vi "Solve Tridiagonal Equations (multiple right hand DBL).vi"(8 "Known Matrix":T1, 9 "Pivot":i32[](array[numeric]), 10 "U":T2, 11 "L":dbl[](array[numeric])) -> (0 "error":i32, 3 "Solution Matrix":T1)   [LabVIEW 2020, in "NI_AALPro.lvlib"]
uses:
  NI_AALPro.lvlib
  RealMatrix.ctl
  <resource>/lvanlys.dll
  NI_Matrix.lvlib
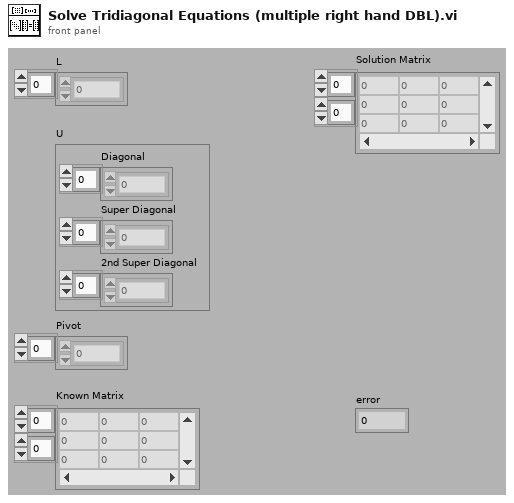
[diagram p1: front panel]
types:
  T1 = typedef "NI_Matrix.lvlib/RealMatrix.ctl" = dbl[][]
  T2 = cluster{"Diagonal":dbl[], "Super Diagonal":dbl[], "2nd Super Diagonal":dbl[]}
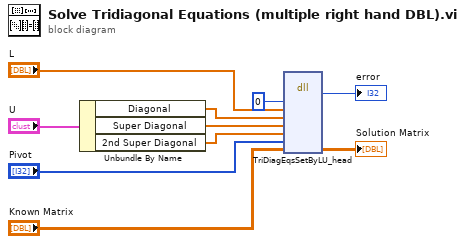
[diagram p0: block diagram]
diagram:
  n1 = Unbundle By Name("U") -> ("Diagonal"=w5:dbl[], "Super Diagonal"=w4:dbl[], "2nd Super Diagonal"=w3:dbl[])
  n2 = dll-call lib="C:/Program Files (x86)/National Instruments/LabVIEW 2020/resource/lvanlys.*" fn="TriDiagEqsSetByLU_head" ("CBLAS.dll:MtrxxVectH")("trans"=0, "L"="L", "Diag"=w5, "SuperDiag"=w4, "SuperDiag2"=w3, "PVT"="Pivot", "B"="Known Matrix") -> ("error"=→"error":i32, "B"=→"Solution Matrix":dbl[][])  [unwired: 9 in, 2 out]
